vi "Count_Up.vi"(11 "Reset?":bool) -> (3 "t":i64)   [LabVIEW 2020]
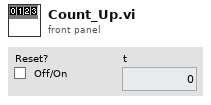
[diagram p1: front panel]
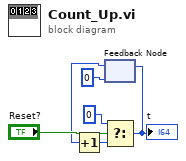
[diagram p0: block diagram]
diagram:
  n1 = feedback #1(i64 0 ("t")) -> (w1:i64)
  n2 = Increment(x=w1) -> (x+1=w2:i64)
  n3 = Select(t=i64 0, s="Reset?", f=w2) -> (s? t:f=w3:i64)
  "t" <- w3
  n4 = feedback-in #1(w3) -> ()
